vi "Dequeue Main Queue & Enqueue Warn&Error.vi"(8 "error in (no error)":errorcluster, 11 "Queue In":refnum<queue>) -> (0 "error out (no error)":errorcluster, 2 "Main Loop State":T1=enum."Initialize", 3 "Queue Out":refnum<queue>, 5 "Parameter":string, 7 "Variant":variant)   [LabVIEW 2019]
uses:
  Type Definitions/Main Loop States.ctl
  Type Definitions/Main Loop Queue Data.ctl
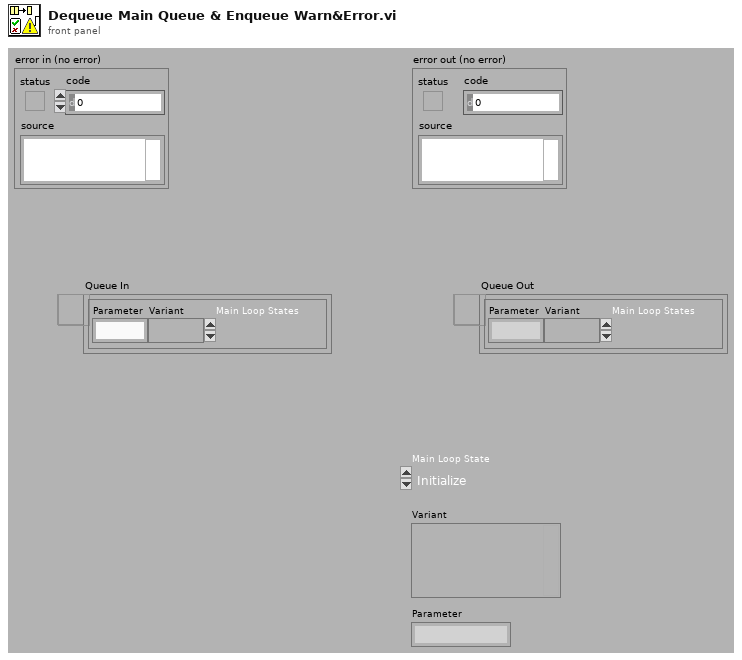
[diagram p1: front panel]
types:
  T1 = typedef "Main Loop States.ctl" = enum16{"  -----  Core  -----  ", "Blank", "Idle", "Initialize", "Shutdown", "Error", "  ----- meerstetter TEC Functions -----  ", "TE Controller"}
  T2 = typedef "Main Loop Queue Data.ctl" = cluster{"Parameter":string, "Variant":variant, "Main Loop States":T1}
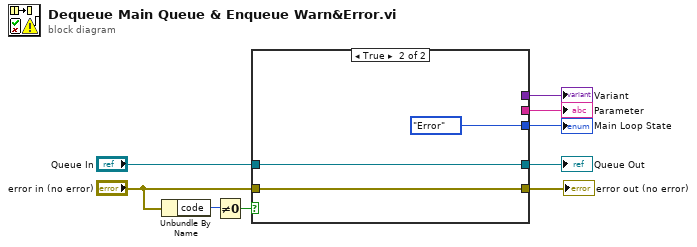
[diagram p0: block diagram]
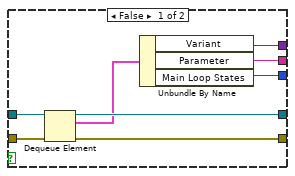
[diagram p2: hidden frame]
diagram:
  n1 = Unbundle By Name("error in (no error)") -> ("code"=w7:i32)
  n2 = Not Equal To 0?(x=w7) -> (x != 0?=w6:bool)
  n3 = case shown="True" w6 {
    tunnel: "Queue In" -> [w17 w20]
    tunnel: [w16 w19] -> w5
    tunnel: [w15 w20] -> w9
    tunnel: "error in (no error)" -> [w14 w19]
    tunnel: [w12 Main_Loop_States."Error" ("Main Loop States")] -> w3
    tunnel: [w11 _] -> w1
    tunnel: [w10 _] -> w2
    frame False {
      n4 = Dequeue Element(queue=w17, error in (no error)=w14) -> (queue out=w15:refnum<queue>, element=w13:T2, error out=w16:errorcluster)  [unwired: 1 in, 1 out]
      n5 = Unbundle By Name(w13) -> ("Variant"=w11:variant, "Parameter"=w10:string, "Main Loop States"=w12:T1)
    }
    frame True {
    }
  }
  "Queue Out" <- w9
  "error out (no error)" <- w5
  "Main Loop State" <- w3
  "Parameter" <- w2
  "Variant" <- w1
